vi "Set_state.vi"(8 "error in (no error)":errorcluster, 10 "States":T1, 11 "MotionModule runtime_in":refnum<class "MotionModule runtime.lvclass">) -> (0 "error out":errorcluster, 3 "MotionModule runtime_out":refnum<class "MotionModule runtime.lvclass">)   [LabVIEW 2017, in "MotionModule runtime.lvclass"]
uses:
  MotionModule runtime.lvclass
  Utilities/StateMachine.ctl
  MotionModule runtime.lvclass/MotionModule runtime.ctl
  Utilities/WordManipulationLibrary.lvlib
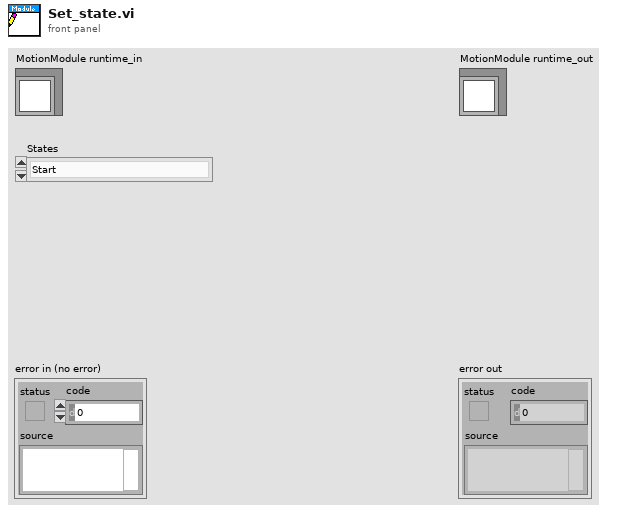
[diagram p1: front panel]
types:
  T1 = typedef "WordManipulationLibrary.lvlib/StateMachine.ctl" = enum16{"Start", "Not Ready to Switch On", "Switch On Disabled", "Ready to Switch On", "Switched On", "Operation enable", "Quick Stop Active", "Fault Reaction Active", "Fault"}
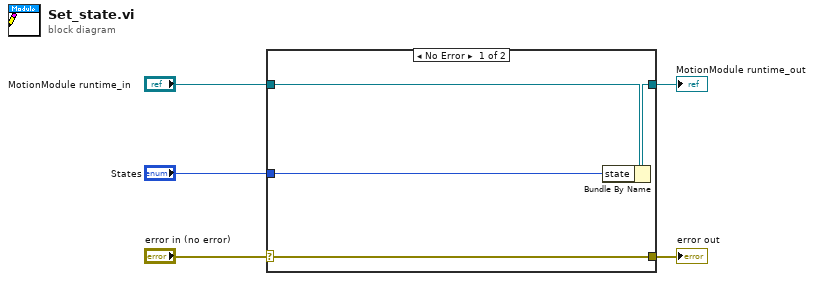
[diagram p0: block diagram]
diagram:
  n1 = case shown="No Error" "error in (no error)" {
    selector: "error in (no error)" -> [w9 w10]
    tunnel: [w9 w10] -> w4
    tunnel: [w7 w11] -> w2
    tunnel: "MotionModule runtime_in" -> [w8 w11]
    tunnel: "States" -> [w6 _]
    frame No Error {
      n2 = Bundle By Name(cluster=w8, "state"=w6) -> (w7:refnum<class "MotionModule runtime.lvclass">)
    }
    frame Error {
    }
  }
  "error out" <- w4
  "MotionModule runtime_out" <- w2
